vi "ALARM Check Sens.vi"(8 "error in (no error)":errorcluster, 10 "Sens Status Old":dbl[](array[numeric]), 11 "register values":dbl[][](array[numeric])) -> (0 "error out":errorcluster, 3 "Sens Status New":i16[](array[numeric]))   [LabVIEW 2020, in "QCT ALARM.lvlib"]
uses:
  QCT ALARM.lvlib
panel:
  out "Waveform Graph":dbl[](graph)
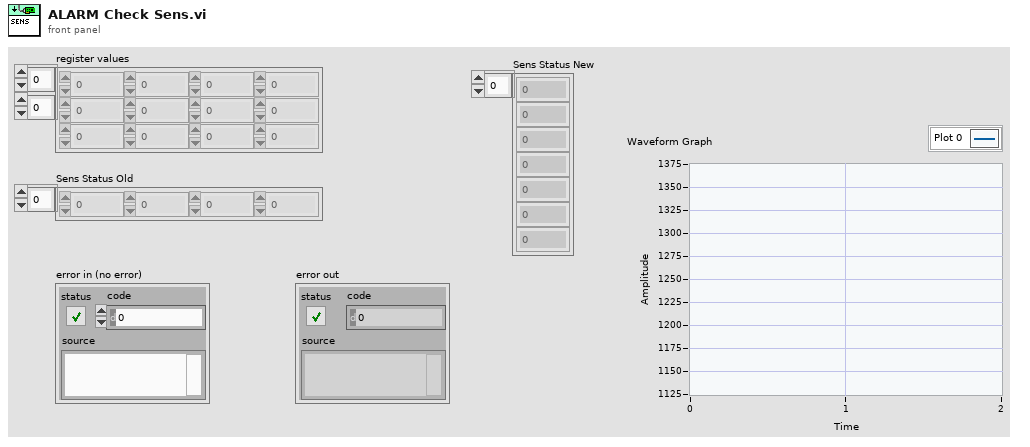
[diagram p1: front panel]
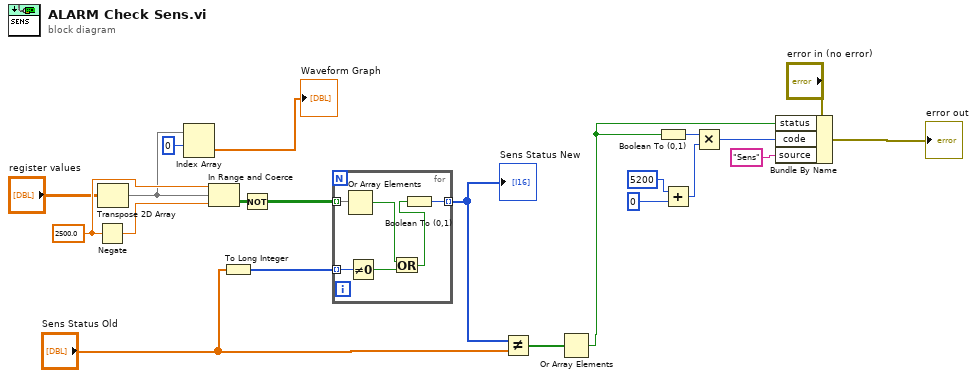
[diagram p0: block diagram]
diagram:
  w18 = 2500.0 ("Threshold")
  n1 = Negate(x=w18) -> (-x=w17:dbl)
  n2 = Transpose 2D Array(2D array="register values") -> (transposed array=w4:dbl[][])
  n3 = Index Array(array=w4, index (row)=0) -> (element=→"Waveform Graph":dbl[])  [unwired: 1 in]
  n4 = In Range and Coerce(upper limit=w18, x=w4, lower limit=w17) -> (In Range?=w5:bool[][])  [unwired: 1 out]
  n5 = To Long Integer(number="Sens Status Old") -> (32bit integer=w6:i32[])
  n6 = Not(x=w5) -> (.not. x?=w21:bool[][])
  n7 = for {
    tunnel: [w27] -> w19 mode=indexing
    tunnel: w21 -> [w23] mode=indexing
    tunnel: w6 -> [w25] mode=indexing
    n8 = Or Array Elements(Boolean array=w23) -> (logical OR=w22:bool)
    n9 = Not Equal To 0?(x=w25) -> (x != 0?=w26:bool)
    n10 = Or(x=w22, y=w26) -> (x .or. y?=w24:bool)
    n11 = Boolean To (0,1)(Boolean=w24) -> (0, 1=w27:i16)
  }
  "Sens Status New" <- w19
  n12 = Not Equal?(x=w19, y="Sens Status Old") -> (x != y?=w20:bool[])
  n13 = Or Array Elements(Boolean array=w20) -> (logical OR=w1:bool)
  n14 = Boolean To (0,1)(Boolean=w1) -> (0, 1=w15:i16)
  n15 = Add(x=5200 ("code"), y=0) -> (x+y=w13:i32)
  n16 = Multiply(x=w15, y=w13) -> (x*y=w14:i32)
  n17 = Bundle By Name(cluster="error in (no error)", "status"=w1, "code"=w14, "source"="Sens") -> (→"error out":errorcluster)
